vi "NMLWSD_FGV.vi"(6 "SysTrue Write":bool[][](array[boolean]), 7 "MCUTrue Write":bool[][](array[boolean]), 8 "Action":enum16{"Initialize", "Read", "Write"}(ring), 9 "FW PRM Count":i32=1 min=1 max=8 step=1, 10 "UUT Count":i32=1 min=1 max=8 step=1, 11 "Points Write":i32[](array[numeric])) -> (0 "SysTrue":bool[][](array[boolean]), 1 "MCUTrue":bool[][](array[boolean]), 3 "Points Read":i32[](array[numeric]))   [LabVIEW 2017]
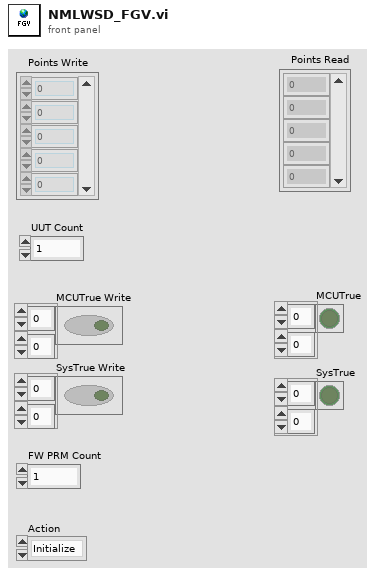
[diagram p1: front panel]
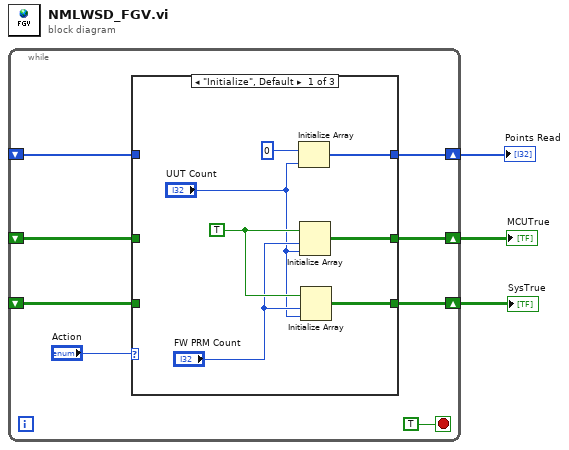
[diagram p0: block diagram]
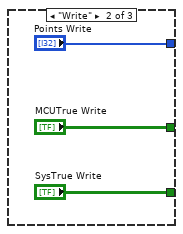
[diagram p2: hidden frame]
diagram:
  n1 = while {
    shift-right: [w9] -> w3
    shift-left: _ -> [w8]
    shift-right: [w7] -> w2
    shift-left: _ -> [w5]
    shift-right: [w6] -> w1
    shift-left: _ -> [w4]
    stop <- TRUE stop-if-true
    n2 = case shown="\"Initialize\", Default" "Action" {
      tunnel: [w18 "Points Write" w24] -> w9
      tunnel: w8 -> [_ _ w24]
      tunnel: [w15 "MCUTrue Write" w23] -> w7
      tunnel: [w14 "SysTrue Write" w22] -> w6
      tunnel: w5 -> [_ _ w23]
      tunnel: w4 -> [_ _ w22]
      frame "Initialize", Default {
        w16 = TRUE
        n3 = Initialize Array(0 ("element"), "UUT Count") -> (w18:i32[])
        n4 = Initialize Array(w16, "FW PRM Count", "UUT Count") -> (w15:bool[][])
        n5 = Initialize Array(w16, "FW PRM Count", "UUT Count") -> (w14:bool[][])
      }
      frame "Write" {
      }
      frame "Read" {
      }
    }
  }
  "Points Read" <- w3
  "MCUTrue" <- w2
  "SysTrue" <- w1
